vi "Assignment2_2.vi"() -> ()   [LabVIEW 2025]
uses:
  TypeDef/Cluster1.ctl
panel:
  out "Valid_Upto_Search_Result":T1[](array[typedef])
  out "Card_Number_Search_Result":T1[](array[typedef])
  out "Card_Holder_Name_Search_Result":T1[](array[typedef])
  out "Search_Time(ms)":dbl
  in  "Search_Option":T2(ring)
  in  "Valid Upto":dbl
  in  "Card Number":dbl
  in  "Card Holder Name":string
  in  "Account_Details":T1[](array[typedef])=[{"Card_Number"=1.0, "Card_Holder_Name"="Sam ", "Valid_Upto"=2045.0}, {"Card_Number"=2.0, "Card_Holder_Name"="Tom ", "Valid_Upto"=2040.0}, {"Card_Number"=3.0, "Card_Holder_Name"="Jerry ", "Valid_Upto"=2050.0}, {"Card_Number"=4.0, "Card_Holder_Name"="Jack ", "Valid_Upto"=2030.0}]
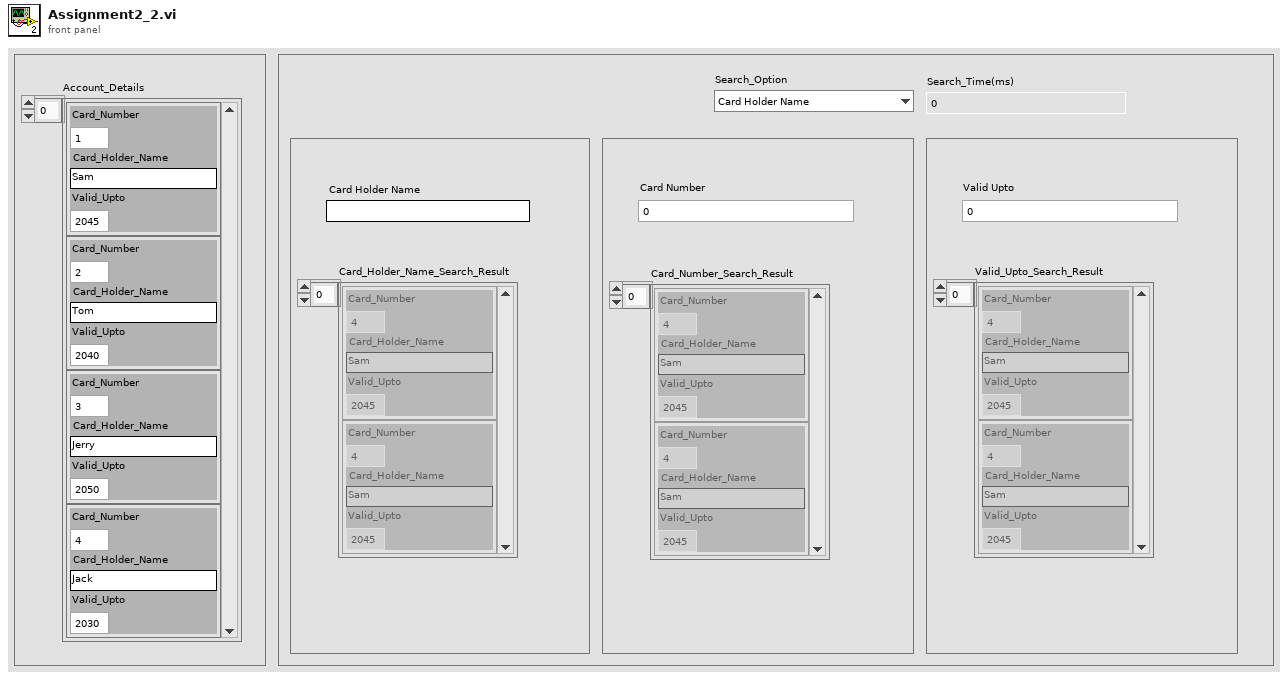
[diagram p1: front panel]
types:
  T1 = typedef "Cluster1.ctl" = cluster{"Card_Number":dbl, "Card_Holder_Name":string, "Valid_Upto":dbl}
  T2 = enum16{"Card Holder Name", "Card Number", "Valid Upto"}
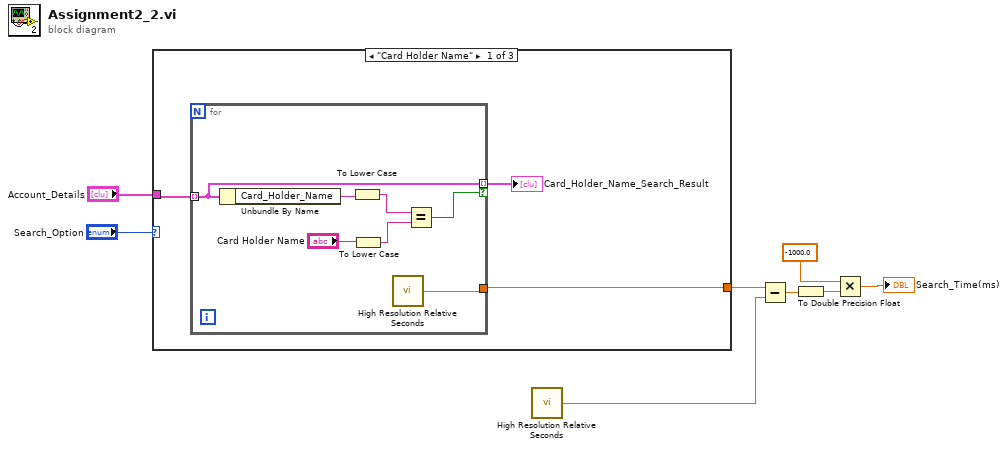
[diagram p0: block diagram]
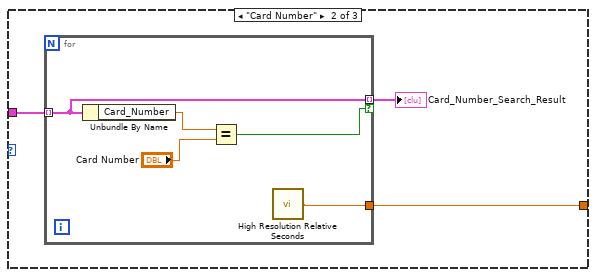
[diagram p2: hidden frame]
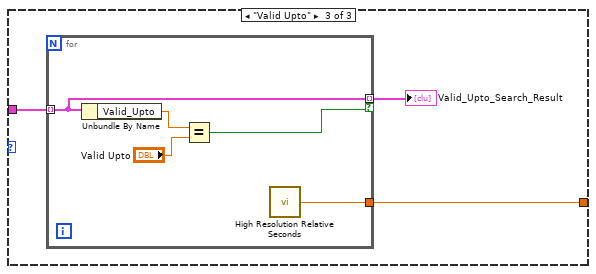
[diagram p3: hidden frame]
diagram:
  n1 = case shown="\"Card Holder Name\"" "Search_Option" {
    tunnel: "Account_Details" -> [w10 w21 w29]
    tunnel: [w9 w19 w27] -> w4
    frame "Card Holder Name" {
      n2 = for {
        tunnel: w10 -> [w14] mode=indexing
        tunnel: [w14] -> w11 mode=indexing if=w13
        tunnel: [w12] -> w9
        n3 = Unbundle By Name(w14) -> ("Card_Holder_Name"=w18:string)
        n4 = To Lower Case(string=w18) -> (all lower case string=w16:string)
        n5 = To Lower Case(string="Card Holder Name") -> (all lower case string=w15:string)
        n6 = call <vilib>:"High Resolution Relative Seconds.vi"() -> ("relative seconds"=w12:dbl)
        n7 = Equal?(x=w16, y=w15) -> (x = y?=w13:bool)
      }
      "Card_Holder_Name_Search_Result" <- w11
    }
    frame "Card Number" {
      n8 = for {
        tunnel: w21 -> [w24] mode=indexing
        tunnel: [w24] -> w20 mode=indexing if=w23
        tunnel: [w22] -> w19
        n9 = Unbundle By Name(w24) -> ("Card_Number"=w26:dbl)
        n10 = Equal?(x=w26, y="Card Number") -> (x = y?=w23:bool)
        n11 = call <vilib>:"High Resolution Relative Seconds.vi"() -> ("relative seconds"=w22:dbl)
      }
      "Card_Number_Search_Result" <- w20
    }
    frame "Valid Upto" {
      n12 = for {
        tunnel: w29 -> [w32] mode=indexing
        tunnel: [w32] -> w28 mode=indexing if=w31
        tunnel: [w30] -> w27
        n13 = Unbundle By Name(w32) -> ("Valid_Upto"=w33:dbl)
        n14 = Equal?(x=w33, y="Valid Upto") -> (x = y?=w31:bool)
        n15 = call <vilib>:"High Resolution Relative Seconds.vi"() -> ("relative seconds"=w30:dbl)
      }
      "Valid_Upto_Search_Result" <- w28
    }
  }
  n16 = call <vilib>:"High Resolution Relative Seconds.vi"() -> ("relative seconds"=w3:dbl)
  n17 = Subtract(x=w4, y=w3) -> (x-y=w6:dbl)
  n18 = To Double Precision Float(number=w6) -> (double precision float=w5:dbl)
  n19 = Multiply(x=-1000.0, y=w5) -> (x*y=→"Search_Time(ms)":dbl)
